vi "LVClass_WavefrontCorrectorSet get plane commands.vi"(0 "WavefrontCorrectorSet in":refnum<class "WavefrontCorrectorSet.lvclass">, 11 "error in (no error)":errorcluster) -> (4 "WavefrontCorrectorSet out":refnum<class "WavefrontCorrectorSet.lvclass">, 6 "PlaneCommand_1D":sgl[](array[numeric]), 15 "error out":errorcluster)   [LabVIEW 2020, in "WavefrontCorrectorSet.lvclass"]
doc: "WavefrontCorrector commands to flat mirror shape getter.\n\n--------------------------------------------------------------------------------\n\n<B>wavefrontcorrector_setIn </B> : WavefrontCorrectorSet object.\n<B>wavefrontcorrector_setOut </B> : WavefrontCorrectorSet object.\n<B>flat_command </B> : Array of commands to apply to have a flat wavefront corrector surface.\n<B>ErrorIn </B> : Error\n<B>ErrorOut </B> : Error\n\n--------------------------------------------------------------------------------"
uses:
  WavefrontCorrectorSet.lvclass
  WavefrontCorrectorSet.lvclass/WavefrontCorrectorSet.ctl
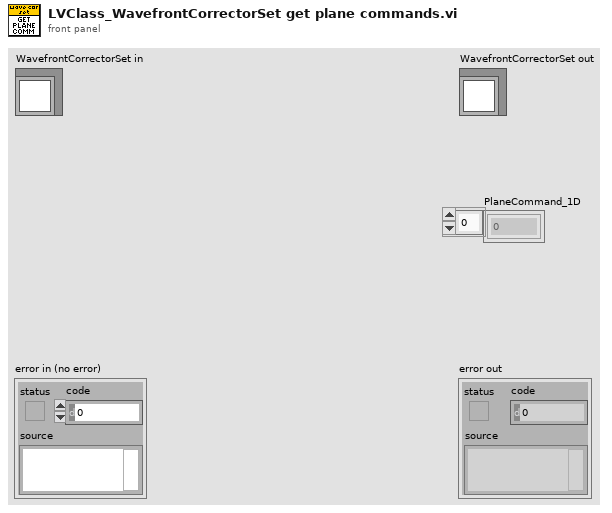
[diagram p1: front panel]
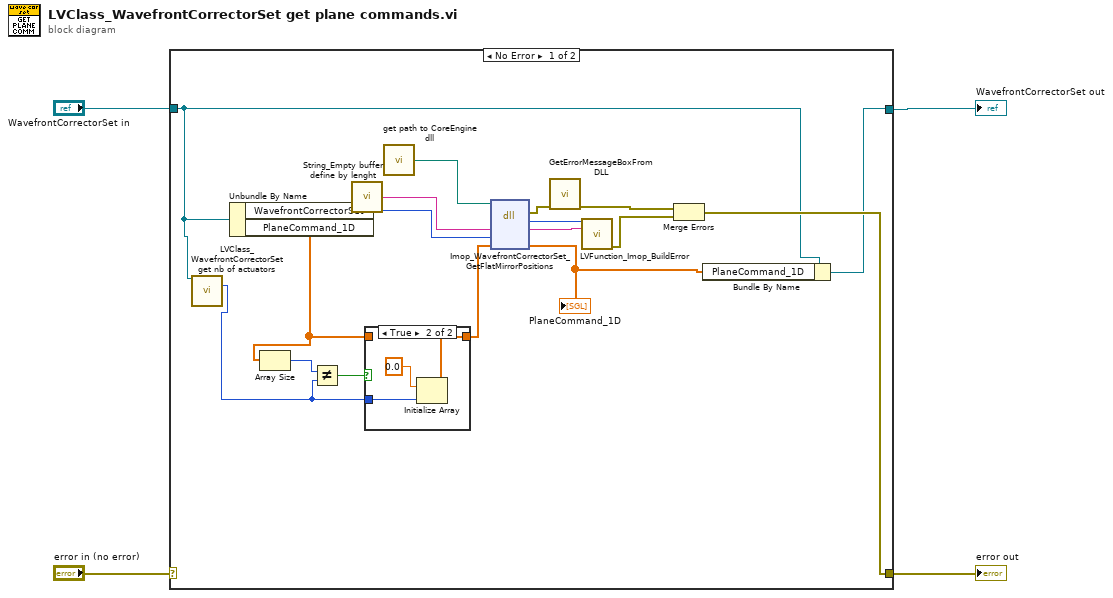
[diagram p0: block diagram]
diagram:
  n1 = case shown="No Error" "error in (no error)" {
    selector: "error in (no error)" -> [_ w27]
    tunnel: [w14 w27] -> w2
    tunnel: [w6 w26] -> w1
    tunnel: "WavefrontCorrectorSet in" -> [w7 w26]
    frame No Error {
      n2 = call "LVClass_WavefrontCorrectorSet get nb of actuators.vi"("WavefrontCorrectorSet in"=w7) -> ("ActuatorsNumber"=w5:i32)  [unwired: 12 in, 2 out]
      n3 = Unbundle By Name(w7) -> ("WavefrontCorrectorSet"=w13:i32, "PlaneCommand_1D"=w10:sgl[])
      n4 = Array Size(array=w10) -> (size(s)=w11:i32)
      n5 = Not Equal?(x=w11, y=w5) -> (x != y?=w12:bool)
      n6 = call "String_Empty buffer define by lenght.vi"() -> ("Empty buffer"=w19:string)  [unwired: 1 in]
      n7 = case shown="True" w12 {
        tunnel: [w22 w24] -> w9
        tunnel: w5 -> [_ w25]
        tunnel: w10 -> [w22 _]
        frame False {
        }
        frame True {
          n8 = Initialize Array(sgl 0.0 ("PlaneCommand_1D"), w25) -> (w24:sgl[])
        }
      }
      n9 = call "get path to CoreEngine dll.vi"() -> ("path to c_interface_vc100.dll"=w18:path)  [unwired: 12 in, 3 out]
      n10 = dll-call lib="D:/soft/HASO_v3/SVN_trunk/ImOpCoreEngine4_LV2011/DLLs/c_interface_vc100.dll" fn="Imop_WavefrontCorrectorSet_GetFlatMirrorPositions"(path in=w18, "message"=w19, "WavefrontCorrectionSet"=w13, "PlaneCommand_1D"=w9) -> (error out=w17:errorcluster, "return type"=w21:i32, "message"=w20:string, "PlaneCommand_1D"=w8:sgl[])  [unwired: 3 in, 1 out]
      "PlaneCommand_1D" <- w8
      n11 = call "GetErrorMessageBoxFromDLL.vi"("error IN"=w17) -> ("error OUT"=w16:errorcluster)  [unwired: 10 in]
      n12 = call "LVFunction_Imop_BuildError.vi"("code"=w21, "String to Prepend to source (\"\")"=w20) -> ("error out"=w15:errorcluster)  [unwired: 13 in]
      n13 = Merge Errors(w16, w15) -> (w14:errorcluster)
      n14 = Bundle By Name(cluster=w7, "PlaneCommand_1D"=w8) -> (w6:refnum<class "WavefrontCorrectorSet.lvclass">)
    }
    frame Error {
    }
  }
  "error out" <- w2
  "WavefrontCorrectorSet out" <- w1
